vi "Poll Button until Pressed.vi"(6 "error in":errorcluster, 8 "polling interval (50 ms)":dbl[unit]=0.05, 9 "button refnum":refnum<vi>) -> (0 "error out":errorcluster, 2 "done":bool)   [LabVIEW 2020]
doc: "This function waits for a button to be pressed or error status is TRUE (error). Polling is performed at a user settable interval (with no timeout)."
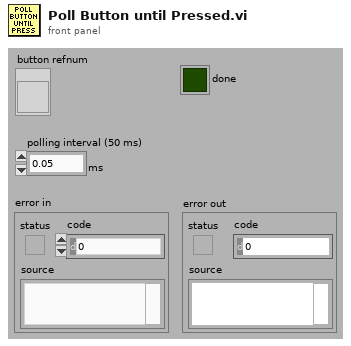
[diagram p1: front panel]
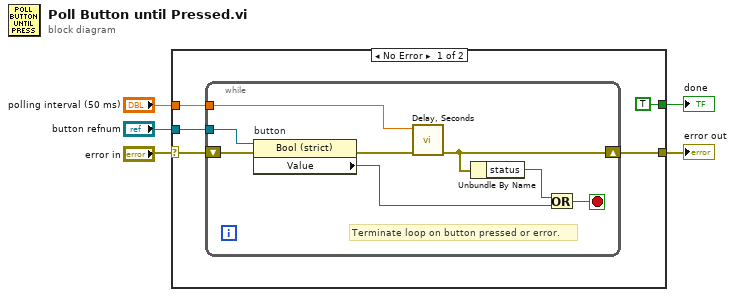
[diagram p0: block diagram]
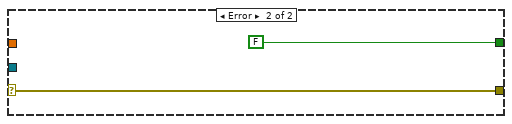
[diagram p2: hidden frame]
diagram:
  n1 = case shown="No Error" "error in" {
    selector: "error in" -> [w10 w20]
    tunnel: [w9 w20] -> w5
    tunnel: [TRUE FALSE] -> w2
    tunnel: "button refnum" -> [w8 _]
    tunnel: "polling interval (50 ms)" -> [w6 _]
    frame No Error {
      n2 = while {
        shift-right: [w13] -> w9
        shift-left: w10 -> [w18]
        tunnel: w8 -> [w12]
        tunnel: w6 -> [w11]
        stop <- w16 stop-if-true
        # "Terminate loop on button pressed or error."
        n3 = property on="button" class="Bool (strict)"(reference=w12, error in=w18) -> (error out=w17:errorcluster, "Value"=w14:bool)  [unwired: 1 out]
        n4 = call "Delay, Seconds.vi"("error in"=w17, "delay"=w11) -> ("error out"=w13:errorcluster)  [unwired: 5 in, 1 out]
        n5 = Unbundle By Name(w13) -> ("status"=w15:bool)
        n6 = Or(x=w15, y=w14) -> (x .or. y?=w16:bool)
      }
    }
    frame Error {
    }
  }
  "error out" <- w5
  "done" <- w2
